vi "ComputeWfmScalar.vi"(6 "GrpCfg":T1, 7 "Speed":T2, 8 "error in (no error)":errorcluster, 10 "Y Array":sgl[](array[numeric]), 11 "Voltage in":refnum<class "Voltage.lvclass">) -> (0 "error out":errorcluster, 2 "Metric":dbl, 3 "Voltage Out":refnum<class "Voltage.lvclass">)   [LabVIEW 2012, in "Measurement Channels.lvlib" / "Voltage.lvclass"]
uses:
  Voltage.lvclass
  Common/Controls/TE_Designator.ctl
  Common/Controls/Group Timing Info.ctl
  <vilib>/addons/_NISVFA/_Shared subVIs/Controls/svc_Window.ctl
  Class Channel/Channel.lvclass
  <vilib>/addons/_NISVFA/_Baseband FFT/SVFA Power Spectrum (1 Ch).vi
  <vilib>/addons/_NISVFA/_Spectrum Processing/SVFA Power in Band (1 Ch).vi
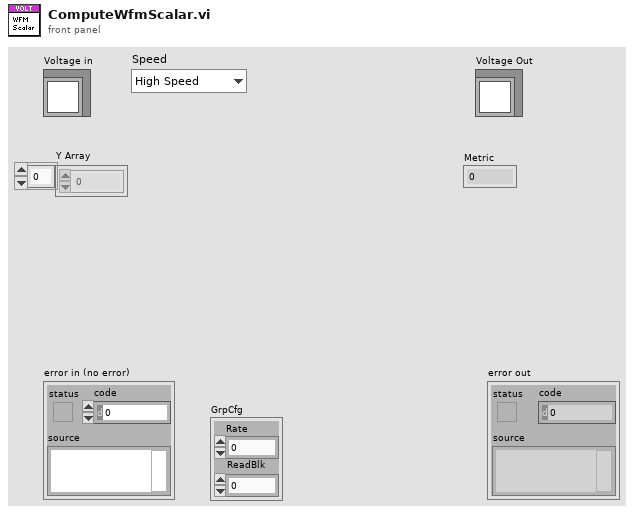
[diagram p1: front panel]
types:
  T1 = typedef "Group Timing Info.ctl" = cluster{"Rate":dbl, "ReadBlk":i32}
  T2 = typedef "TE_Designator.ctl" = enum16{"High Speed", "Low Speed"}
  T3 = typedef "svc_Window.ctl" = u32
  T4 = typedef "svc_Spectrum Info.ctl" = cluster{"channel name":string, "description":string, "x-axis units":T5, "spectral info":cluster{"spectrum type":T6, "linear/dB":enum16{"linear", "dB"}, "window":u16, "window size":i32, "FFT size":i32}, "engineering units":T7, "custom label":string, "dB reference [EU]":dbl, "peak units":enum16{"rms", "peak", "peak-peak"}, "weighting filter":T8, "spectral density?":bool, "unit label":string, "spectrum skewed?":bool, "complimentary spectrum units":T9}
  T5 = typedef "svc_X-Axis Units.ctl" = u16
  T6 = typedef "svc_Spectrum Type.ctl" = enum16{"FFT Spectrum [complex]", "Amplitude [Magnitude]", "Power [Magnitude^2]", "Cross Spectrum [complex]", "Frequency Response [Complex]"}
  T7 = typedef "svc_Engineering Units Text Ring.ctl" = u16
  T8 = typedef "svc_Weighting Filter Text Ring.ctl" = u16
  T9 = typedef "svc_Complimentary Spectrum Units.ctl" = enum16{"none", "radians", "degrees", "cycles", "imaginary"}
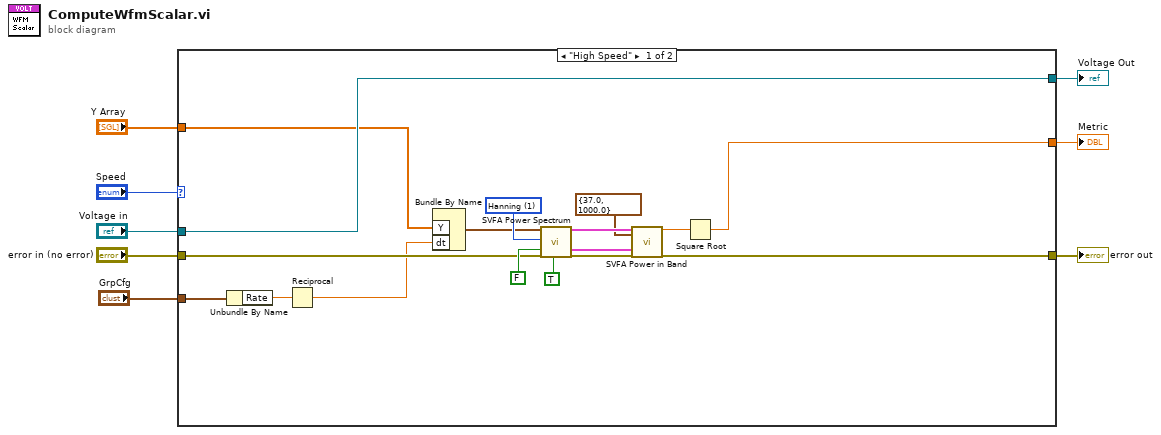
[diagram p0: block diagram]
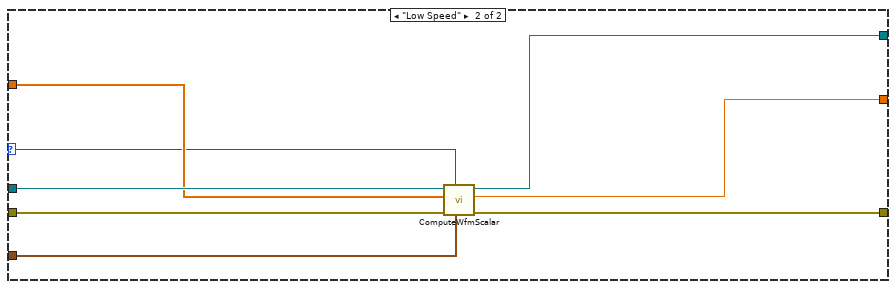
[diagram p2: hidden frame]
diagram:
  n1 = case shown="\"High Speed\"" "Speed" {
    selector: "Speed" -> [_ w29]
    tunnel: "error in (no error)" -> [w14 w32]
    tunnel: "Y Array" -> [w13 w30]
    tunnel: [w18 w27] -> w4
    tunnel: [w16 w31] -> w3
    tunnel: "Voltage in" -> [w15 w33]
    tunnel: [w15 w28] -> w2
    tunnel: "GrpCfg" -> [w11 w26]
    frame "High Speed" {
      w22 = T3 1 items=["None"=0, "Hanning"=1, "Hamming"=2, "Blackman-Harris"=3, "Exact Blackman"=4, "Blackman"=5, "Flat Top"=6, "4 Term B-Harris "=7, "7 Term B-Harris"=8, "Low Sidelobe"=9, "Blackman Nuttall"=11, "Triangle"=30, "Bartlett-Hanning"=31, "Bohman"=32, "Parzen"=33, "Welch"=34, "Kaiser"=60, "Dolph-Chebyshev"=61, "Gaussian"=62] ("window")
      n2 = Unbundle By Name(w11) -> ("Rate"=w10:dbl)
      n3 = Reciprocal(x=w10) -> (1/x=w9:dbl)
      n4 = Bundle By Name("Y"=w13, "dt"=w9) -> (w12:waveform(sgl))  [unwired: 1 in]
      n5 = call-poly <vilib>:"SVFA Power Spectrum.vi"("scaled signal [EU]"=w12, "window"=w22, "dB On (T)"=FALSE, "error in (no error)"=w14, "restart averaging (F)"=TRUE) -> ("power spectrum [dB EU]"=w23:cluster{"f0":dbl, "df":dbl, "magnitude":dbl[]}, "spectrum info"=w25:T4, "error out"=w24:errorcluster)  [unwired: 9 in, 3 out]
      n6 = call-poly <vilib>:"SVFA Power in Band.vi"("spectrum"=w23, "range"=cluster{"start":dbl, "stop":dbl} {"start"=37.0, "stop"=1000.0}, "spectrum info"=w25, "error in (no error)"=w24) -> ("power in band"=w19:dbl, "error out"=w16:errorcluster)  [unwired: 13 in, 1 out]
      n7 = Square Root(x=w19) -> (sqrt(x)=w18:dbl)
    }
    frame "Low Speed" {
      n8 = call-parent "ComputeWfmScalar.vi"("GrpCfg"=w26, "Speed"=w29, "error in (no error)"=w32, "Y Array"=w30, "Channel in"=w33) -> ("error out"=w31:errorcluster, "Metric"=w27:dbl, "Channel Out"=w28:refnum<class "Voltage.lvclass">)  [unwired: 4 in]
    }
  }
  "error out" <- w3
  "Metric" <- w4
  "Voltage Out" <- w2
